vi "Write cost log.vi"(4 "Year":i32, 6 "Month":i32, 7 "Costs in":dbl[](array[numeric]), 8 "error in (no error)":errorcluster, 11 "Refnum in":T1) -> (0 "error out":errorcluster, 3 "Refnum out":T1)   [LabVIEW 2015]
uses:
  <vilib>/Utility/config.llb/Config Data RefNum.ctl
  <vilib>/Utility/config.llb/Read Key (Path).vi
  <vilib>/Utility/file.llb/Write Delimited Spreadsheet (string).vi
  <vilib>/Utility/config.llb/NI_LVConfig.lvlib
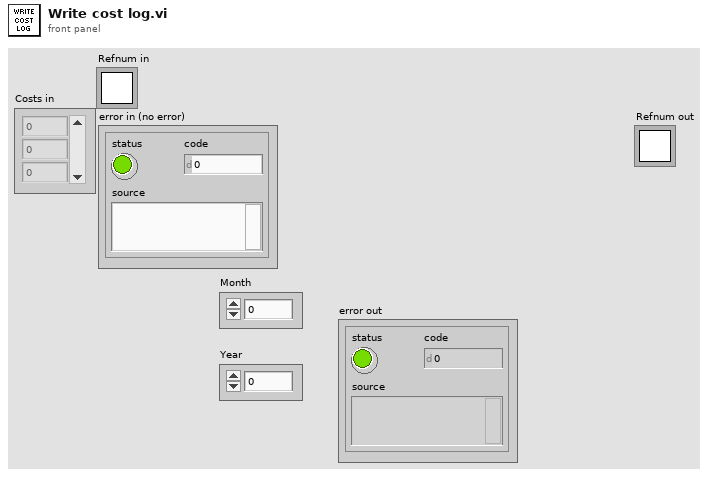
[diagram p1: front panel]
types:
  T1 = typedef "NI_LVConfig.lvlib/Config Data RefNum.ctl" = refnum<k1>
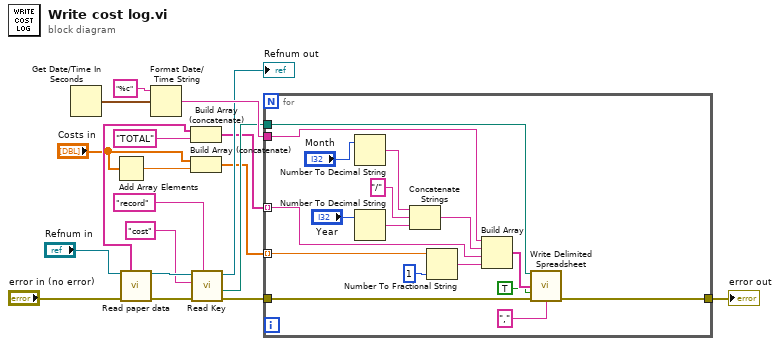
[diagram p0: block diagram]
diagram:
  n1 = Get Date/Time In Seconds() -> (seconds since 1Jan1904=w15:timestamp)
  n2 = Add Array Elements(numeric array="Costs in") -> (sum=w2:dbl)
  n3 = call "Read paper data.vi"("Refnum in"="Refnum in", "error in (no error)"="error in (no error)") -> ("Names"=w12:string[], "Refnum out"=w18:T1, "error out"=w19:errorcluster)  [unwired: 9 in, 2 out]
  n4 = Format Date/Time String(time format string (%c)="%c", seconds (now)=w15) -> (date/time string=w13:string)  [unwired: 1 in]
  n5 = Build Array (concatenate)(w12, "TOTAL" ("element")) -> (w5:string[])
  n6 = Build Array (concatenate)("Costs in", w2) -> (w4:dbl[])
  n7 = call-poly <vilib>:"Read Key.vi"("section"="record", "error in (no error)"=w19, "key"="cost", "refnum"=w18) -> ("error out"=w10:errorcluster, "value"=w11:path, "refnum out"=→"Refnum out":T1)  [unwired: 4 in, 1 out]
  n8 = for {
    tunnel: w13 -> [w34]
    tunnel: w4 -> [w33] mode=indexing
    tunnel: w5 -> [w30] mode=indexing
    tunnel: w11 -> [w29]
    tunnel: w10 -> [w28]
    tunnel: [w25] -> w6
    n9 = Number To Decimal String(number="Month") -> (decimal integer string=w23:string)  [unwired: 1 in]
    n10 = Number To Decimal String(number="Year") -> (decimal integer string=w21:string)  [unwired: 1 in]
    n11 = Concatenate Strings(w23, "/", w21) -> (w20:string)
    n12 = Number To Fractional String(number=w33, precision (6)=i16 1) -> (F-format string=w31:string)  [unwired: 2 in]
    n13 = Build Array(w34, w20, w30, w31) -> (w27:string[])
    n14 = call-poly <vilib>:"Write Delimited Spreadsheet.vi"("file path (dialog if empty)"=w29, "1D data"=w27, "append to file? (F)"=TRUE, "error in (no error)"=w28, "delimiter (\\t)"="," ("delimiter (\\t)")) -> ("error out"=w25:errorcluster)  [unwired: 9 in, 1 out]
  }
  "error out" <- w6
